vi "measVoltGlobVars.vi"() -> ()   [LabVIEW 2014]
uses:
  Controls/measVoltState.ctl
  Controls/measVoltCompleteDest.ctl
panel:
  in  "measVoltCompleteDest":T1
  out "stopVoltMeas":bool caption="measVoltStop"
  in  "measVoltState":T2
  out "timedOutWhileHandshake":bool
  in  "measVoltTimeout(10ns)":i32 caption="measVoltTimeout(25ns)"
  in  "measVoltPulseLength(25ns)":i32
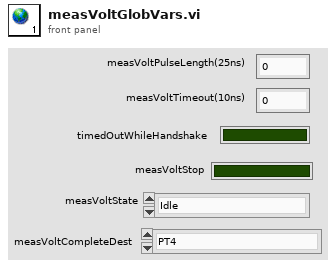
[diagram p1: front panel]
types:
  T1 = typedef "measVoltCompleteDest.ctl" = enum16{"PT4", "C1D30", "C1D31", "PT4_C1D30", "PT4_C1D31", "PT4_C1D30_C1D31", "C1D30_C1D31", "software"}
  T2 = typedef "measVoltState.ctl" = enum16{"Idle", "sendMeasRequest", "waitUntilDone", "done"}
diagram:
